vi "V7310.Main.Status.vi"(8 "error in":errorcluster, 11 "Data in":T1={"Status"={"State"=enum."Init", "LaserStatus"=enum."-", "LaserStatusRaw"="", "Ref"=refnum, "RTC TS"=timestamp(0 s since 1904-01-01), "Conn TS"=timestamp(0 s since 1904-01-01), "Msg"=[], "JobInUse"="", "Jobs"=[], "Vars"=[]}, "Sets"={"Address"="192.168.2.1", "Timeout_ms"=5000, "ReconnectPeriod_s"=0, "JobInUse"="", "CoordinatesOffset"={"X"=0.0, "Y"=0.0}}}) -> (0 "error out":errorcluster, 3 "Data out":T1={"Status"={"State"=enum."Init", "LaserStatus"=enum."-", "LaserStatusRaw"="", "Ref"=refnum, "RTC TS"=timestamp(0 s since 1904-01-01), "Conn TS"=timestamp(0 s since 1904-01-01), "Msg"=[], "JobInUse"="", "Jobs"=[], "Vars"=[]}, "Sets"={"Address"="192.168.2.1", "Timeout_ms"=5000, "ReconnectPeriod_s"=0, "JobInUse"="", "CoordinatesOffset"={"X"=0.0, "Y"=0.0}}})   [LabVIEW 2016]
uses:
  V7310.Data.ctl
  V7310.Data.Status.ctl
  V7310.Data.Status.State.ctl
  LowLevel/V7310.LaserStatus.ctl
  LowLevel/V7310.Message.Data.ctl
  LowLevel/V7310.Job.Variable.ctl
  V7310.Data.Sets.ctl
  tools/EventLog/EventLog.EventSource.ctl
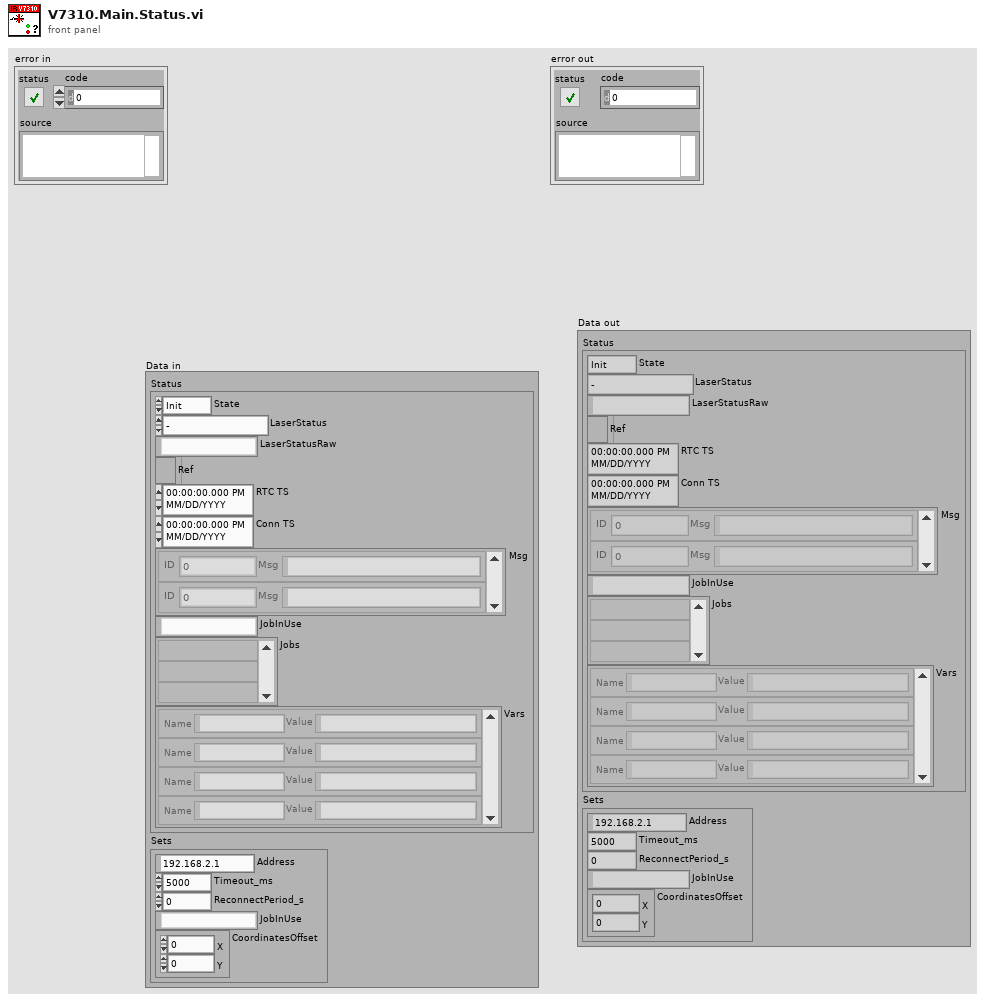
[diagram p1: front panel]
types:
  T1 = typedef "V7310.Data.ctl" = cluster{"Status":T2, "Sets":T7}
  T2 = typedef "V7310.Data.Status.ctl" = cluster{"State":T3, "LaserStatus":T4, "LaserStatusRaw":string, "Ref":refnum<k5>, "RTC TS":timestamp, "Conn TS":timestamp, "Msg":T5[], "JobInUse":string, "Jobs":string[], "Vars":T6[]}
  T3 = typedef "V7310.Data.Status.State.ctl" = enum16{"First", "Init", "Msg", "Error", "Abort", "Idle", "Run"}
  T4 = typedef "V7310.LaserStatus.ctl" = enum16{"-", "FatalError", "Initialize", "KeySwitchOpen", "TimeoutInterlock", "InterlockOpen", "StartUp", "ShutterlockOpen", "Standby", "Ready", "PrepareForMarking", "WaitForTrigger", "Marking"}
  T5 = typedef "V7310.Message.Data.ctl" = cluster{"ID":i32, "Msg":string}
  T6 = typedef "V7310.Job.Variable.ctl" = cluster{"Name":string, "Value":string}
  T7 = typedef "V7310.Data.Sets.ctl" = cluster{"Address":string, "Timeout_ms":i32, "ReconnectPeriod_s":i32, "JobInUse":string, "CoordinatesOffset":cluster{"X":dbl, "Y":dbl}}
  T8 = typedef "EventLog.EventSource.ctl" = enum16{"All", "Gui", "Ref", "File", "Arch", "Seq", "CPX", "DB", "Laser", "Scan.P", "Scan.O"}
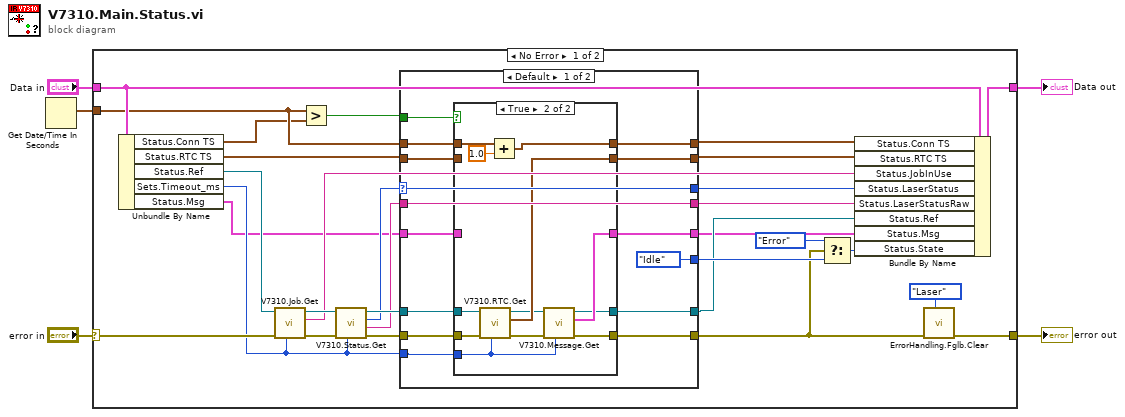
[diagram p0: block diagram]
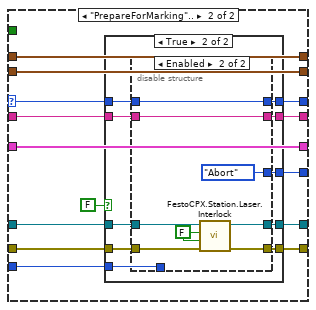
[diagram p3: hidden frame]
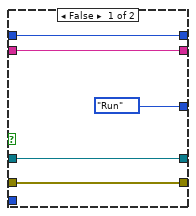
[diagram p4: hidden frame]
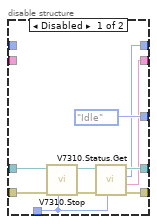
[diagram p5: hidden frame]
diagram:
  n1 = Get Date/Time In Seconds() -> (seconds since 1Jan1904=w1:timestamp)
  n2 = case shown="No Error" "error in" {
    selector: "error in" -> [w15 w114]
    tunnel: [w29 w114] -> w2
    tunnel: "Data in" -> [w31 w113]
    tunnel: [w34 w113] -> w3
    tunnel: w1 -> [w10 _]
    frame No Error {
      n3 = Unbundle By Name(w31) -> ("Status.Conn TS"=w9:timestamp, "Status.RTC TS"=w16:timestamp, "Status.Ref"=w11:refnum<k5>, "Sets.Timeout_ms"=w12:i32, "Status.Msg"=w6:T5[])
      n4 = call "V7310.Job.Get.vi"("timeout ms (5000)"=w12, "error in"=w15, "Connection in"=w11) -> ("error out"=w14:errorcluster, "Job"=w7:string, "Connection out"=w13:refnum<k5>)  [unwired: 6 in]
      n5 = Greater?(x=w10, y=w9) -> (0:w19:bool)
      n6 = call "V7310.Status.Get.vi"("timeout ms (5000)"=w12, "error in"=w14, "Connection in"=w13) -> ("error out"=w27:errorcluster, "Laser Status"=w23:string, "LaserStatus"=w24:T4, "Connection out"=w26:refnum<k5>)  [unwired: 5 in]
      n7 = case shown="Default" w24 {
        selector: w24 -> [w36 w69]
        tunnel: [V7310.Data.Status.State."Idle" ("Status.State") w72] -> w28
        tunnel: w27 -> [w46 w80]
        tunnel: [w43 w78] -> w22
        tunnel: w26 -> [w45 w79]
        tunnel: [w44 w77] -> w21
        tunnel: w12 -> [w42 w76]
        tunnel: [w36 w75] -> w8
        tunnel: [w48 w74] -> w25
        tunnel: w23 -> [w48 w73]
        tunnel: [w47 w68] -> w20
        tunnel: w19 -> [w41 _]
        tunnel: w10 -> [w40 w70]
        tunnel: [w39 w71] -> w18
        tunnel: [w38 w70] -> w17
        tunnel: w16 -> [w37 w71]
        tunnel: w6 -> [w35 w68]
        frame Default {
          n8 = case shown="True" w41 {
            tunnel: [w54 w66] -> w43
            tunnel: [w50 w65] -> w47
            tunnel: w46 -> [w54 w64]
            tunnel: w45 -> [w53 w63]
            tunnel: w42 -> [_ w62]
            tunnel: [w51 w61] -> w39
            tunnel: [w53 w60] -> w44
            tunnel: w40 -> [w52 w59]
            tunnel: [w52 w57] -> w38
            tunnel: w37 -> [w51 _]
            tunnel: w35 -> [w50 _]
            frame False {
            }
            frame True {
              n9 = call "V7310.RTC.Get.vi"("timeout ms (5000)"=w62, "error in"=w64, "Connection in"=w63) -> ("error out"=w56:errorcluster, "RTC"=w61:timestamp, "Connection out"=w55:refnum<k5>)  [unwired: 5 in, 1 out]
              n10 = Add(x=w59, y=1.0) -> (x+y=w57:timestamp)
              n11 = call "V7310.Message.Get.vi"("timeout ms (5000)"=w62, "error in"=w56, "Connection in"=w55) -> ("error out"=w66:errorcluster, "Messages"=w65:T5[], "Connection out"=w60:refnum<k5>)  [unwired: 6 in]
            }
          }
        }
        frame "PrepareForMarking".. {
          n12 = case shown="True" FALSE {
            tunnel: w80 -> [w84 w95]
            tunnel: w79 -> [w83 w94]
            tunnel: [V7310.Data.Status.State."Run" ("Status.State") w93] -> w72
            tunnel: [w84 w90] -> w78
            tunnel: [w83 w91] -> w77
            tunnel: w76 -> [_ w92]
            tunnel: [w82 w89] -> w75
            tunnel: [w81 w88] -> w74
            tunnel: w69 -> [w82 w87]
            tunnel: w73 -> [w81 w86]
            frame False {
            }
            frame True {
              n13 = disable-structure shown="Enabled" {
                disable-tunnel: w95 -> [w105 w109]
                disable-tunnel: w94 -> [w104 w107]
                disable-tunnel: [V7310.Data.Status.State."Idle" ("Status.State") V7310.Data.Status.State."Abort" ("Status.State")] -> w93
                disable-tunnel: w92 -> [w100 _]
                disable-tunnel: [w99 w107] -> w91
                disable-tunnel: [w98 w108] -> w90
                disable-tunnel: [w97 w112] -> w89
                disable-tunnel: [w96 w111] -> w88
                disable-tunnel: w87 -> [_ w112]
                disable-tunnel: w86 -> [_ w111]
                frame Disabled {
                  n14 = call "V7310.Stop.vi"("timeout ms (5000)"=w100, "error in"=w105, "Connection in"=w104) -> ("error out"=w101:errorcluster, "Connection out"=w102:refnum<k5>)  [unwired: 7 in]
                  n15 = call "V7310.Status.Get.vi"("timeout ms (5000)"=w100, "error in"=w101, "Connection in"=w102) -> ("error out"=w98:errorcluster, "Laser Status"=w96:string, "LaserStatus"=w97:T4, "Connection out"=w99:refnum<k5>)  [unwired: 5 in]
                }
                frame Enabled {
                  w106 = FALSE ("Shutterlock")
                  n16 = call "FestoCPX.Station.Laser.Interlock.vi"("error in"=w109, "Wait (T)"=w106, "Interlock"=w106) -> ("error out"=w108:errorcluster)  [unwired: 8 in]
                }
              }
            }
          }
        }
      }
      n17 = Select(t=V7310.Data.Status.State."Error" ("Status.State"), s=w22, f=w28) -> (s? t:f=w32:T3)
      n18 = Bundle By Name(cluster=w31, "Status.Conn TS"=w17, "Status.RTC TS"=w18, "Status.JobInUse"=w7, "Status.LaserStatus"=w8, "Status.LaserStatusRaw"=w25, "Status.Ref"=w21, "Status.Msg"=w20, "Status.State"=w32) -> (w34:T1)
      n19 = call "ErrorHandling.Fglb.Clear.vi"("Event source"=EventLog.EventSource."Laser", "error in (no error)"=w22) -> ("error out"=w29:errorcluster)  [unwired: 9 in]
    }
    frame Error {
    }
  }
  "error out" <- w2
  "Data out" <- w3
